vi "Draw Overlay.vi"(0 "Image (in)":T1, 1 "Image Width (in)":i32, 2 "Image Height (in)":i32, 3 "X Center (in)":sgl[](array[numeric]), 4 "Y Center (in)":sgl[](array[numeric]), 5 "Height (in)":sgl[](array[numeric]), 6 "Colors (in)":u32[](array[numeric]), 7 "Width (in)":sgl[](array[numeric]), 8 "Classes (in)":i32[](array[numeric]), 9 "Orienation (in)":sgl[](array[numeric])) -> (14 "Image (out)":T1)   [LabVIEW 2016]
uses:
  <vilib>/vision/Image Controls.llb/IMAQ Image.ctl
  <vilib>/Analysis/coordinate.llb/2D Cartesian Coordinate Rotation (Array).vi
  <vilib>/Analysis/NI_AALPro.lvlib
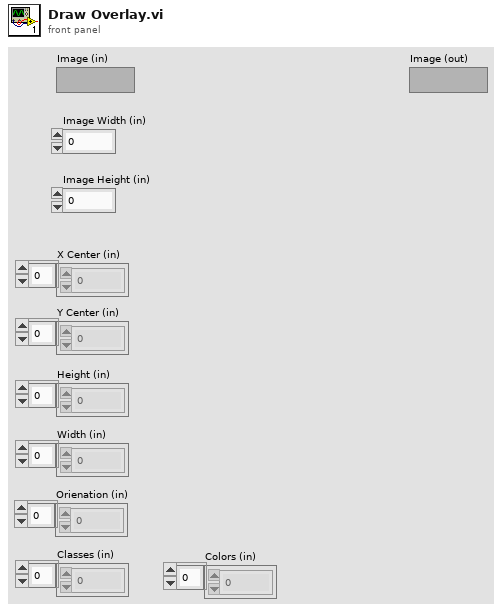
[diagram p1: front panel]
types:
  T1 = typedef "IMAQ Image.ctl" = refnum<image>
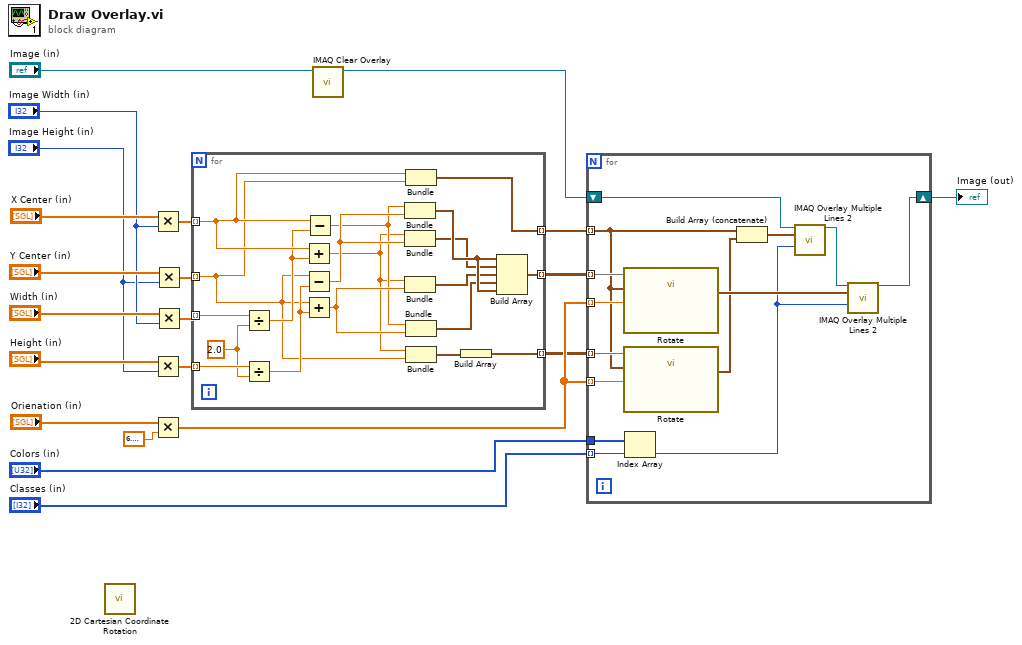
[diagram p0: block diagram]
diagram:
  n1 = call-poly <vilib>:"2D Cartesian Coordinate Rotation.vi"() -> ()  [unwired: 9 in, 3 out]
  n2 = Multiply(x="X Center (in)", y="Image Width (in)") -> (x*y=w9:sgl[])
  n3 = Multiply(x="Height (in)", y="Image Height (in)") -> (x*y=w12:sgl[])
  n4 = Multiply(x="Orienation (in)", y=6.283185307179586) -> (x*y=w2:dbl[])
  n5 = Multiply(x="Y Center (in)", y="Image Height (in)") -> (x*y=w10:sgl[])
  n6 = Multiply(x="Width (in)", y="Image Width (in)") -> (x*y=w11:sgl[])
  n7 = for {
    tunnel: w9 -> [w29] mode=indexing
    tunnel: w10 -> [w22] mode=indexing
    tunnel: w11 -> [w36] mode=indexing
    tunnel: w12 -> [w35] mode=indexing
    tunnel: [w30] -> w6 mode=indexing
    tunnel: [w28] -> w5 mode=indexing
    tunnel: [w25] -> w1 mode=indexing
    w34 = 2.0
    n8 = Divide(x=w36, y=w34) -> (x/y=w27:dbl)
    n9 = Divide(x=w35, y=w34) -> (x/y=w23:dbl)
    n10 = Add(x=w29, y=w27) -> (x+y=w24:dbl)
    n11 = Subtract(x=w22, y=w23) -> (x-y=w33:dbl)
    n12 = Add(x=w22, y=w23) -> (x+y=w32:dbl)
    n13 = Subtract(x=w29, y=w27) -> (x-y=w31:dbl)
    n14 = Bundle(w31, w33) -> (w40:cluster{dbl, dbl})  [unwired: 1 in]
    n15 = Bundle(w24, w33) -> (w37:cluster{dbl, dbl})  [unwired: 1 in]
    n16 = Bundle(w24, w32) -> (w38:cluster{dbl, dbl})  [unwired: 1 in]
    n17 = Bundle(w29, w22) -> (w28:cluster{sgl, sgl})  [unwired: 1 in]
    n18 = Bundle(w31, w32) -> (w39:cluster{dbl, dbl})  [unwired: 1 in]
    n19 = Bundle(w24, w22) -> (w26:cluster{dbl, sgl})  [unwired: 1 in]
    n20 = Build Array(w26) -> (w25:cluster{dbl, sgl}[])
    n21 = Build Array(w40, w37, w38, w39, w40) -> (w30:cluster{dbl, dbl}[])
  }
  n22 = call "IMAQ Clear Overlay"("Image"="Image (in)") -> ("Image Out"=w21:T1)  [unwired: 9 in, 1 out]
  n23 = for {
    shift-right: [w54] -> w8
    shift-left: w21 -> [w46]
    tunnel: "Classes (in)" -> [w53] mode=indexing
    tunnel: "Colors (in)" -> [w52]
    tunnel: w6 -> [w51] mode=indexing
    tunnel: w5 -> [w45] mode=indexing
    tunnel: w2 -> [w50] mode=indexing
    tunnel: w2 -> [w48] mode=indexing
    tunnel: w1 -> [w47] mode=indexing
    n24 = call "Rotate.vi"("Theta (Radians)"=w50, "Pivot Point"=w45, "Points to Rotate"=w51) -> ("Rotated Points"=w49:cluster{"x out":dbl, "y out":dbl}[])  [unwired: 8 in]
    n25 = call "Rotate.vi"("Theta (Radians)"=w48, "Pivot Point"=w45, "Points to Rotate"=w47) -> ("Rotated Points"=w44:cluster{"x out":dbl, "y out":dbl}[])  [unwired: 8 in]
    n26 = Index Array(array=w52, index=w53) -> (element=w41:u32)
    n27 = Build Array (concatenate)(w45, w44) -> (w43:cluster{"x out":dbl, "y out":dbl}[])
    n28 = call "IMAQ Overlay Multiple Lines 2"("Image"=w46, "Line End Points"=w43, "Color"=w41) -> ("Image Out"=w42:T1)  [unwired: 11 in, 1 out]
    n29 = call "IMAQ Overlay Multiple Lines 2"("Image"=w42, "Line End Points"=w49, "Color"=w41) -> ("Image Out"=w54:T1)  [unwired: 11 in, 1 out]
  }
  "Image (out)" <- w8
